vi "Write With Abort.vi"(6 "abort":bool, 10 "element":T1) -> (2 "channel":T2, 4 "aborted?":bool, 5 "previous element":T1)   [LabVIEW 2020]
doc: "Writes a value to a Tag channel or signals the channel to abort. This endpoint is the same as the Write endpoint except that it has an <B>abort</B> input and an <B>aborted?</B> output. You can use the abort capability of the Tag channel to close a channel abruptly, ignoring any data left in the channel buffer. You must use this endpoint together with the Read With Abort endpoint."
uses:
  Element.ctl
  Flex.lvlib
  ))Channel.ctl
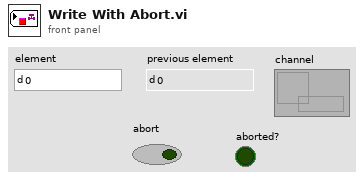
[diagram p1: front panel]
types:
  T1 = typedef "Flex.lvlib/Element.ctl" = dbl
  T2 = typedef "Flex.lvlib/))Channel.ctl" = refnum<queue>
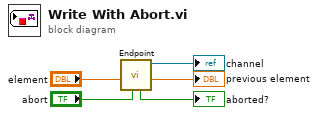
[diagram p0: block diagram]
diagram:
  n1 = call "Endpoint.vi"("abort (F)"="abort", "element in"="element") -> ("element out"=→"previous element":T1, "channel out"=→"channel":T2, "aborted?"=→"aborted?":bool)  [unwired: 6 in, 1 out]
